vi "K2450 Ramp Current.vi"() -> ()   [LabVIEW 2025]
doc: "Author: Scott Hannahs <sth@magnet.fsu.edu>\n\nThis software is licensed for use under the “MIT License\"\nCopyright (c) 2025 Scott Hannahs, sth@sth@magnet.sthnet.net\n\nPermission is hereby granted, free of charge, to any person obtaining a copy of this software and associated documentation files (the \"Software\"), to deal in the Software without restriction, including without limitation the rights to use, copy, modify, merge, publish, distribute, sublicense, and/or sell copies of the Software, and to permit persons to whom the Software is furnished to do so, subject to the following conditions: The above copyright notice and this permission notice shall be included in all copies or substantial portions of the Software.\n\nTHE SOFTWARE IS PROVIDED \"AS IS\", WITHOUT WARRANTY OF ANY KIND, EXPRESS OR IMPLIED, INCLUDING BUT NOT LIMITED TO THE WARRANTIES OF MERCHANTABILITY, FITNESS FOR A PARTICULAR PURPOSE AND NONINFRINGEMENT. IN NO EVENT SHALL THE AUTHORS OR COPYRIGHT HOLDERS BE LIABLE FOR ANY CLAIM, DAMAGES OR OTHER LIABILITY, WHETHER IN AN ACTION OF CONTRACT, TORT OR OTHERWISE, ARISING FROM, OUT OF OR IN CONNECTION WITH THE SOFTWARE OR THE USE OR OTHER DEALINGS IN THE SOFTWARE."
panel:
  out "Time Remaining":dbl=60.0 format="%<%H:%M:%S>t"
  out "Output Current":dbl format="%_4g"
  in  "Time (Hr:Min:Sec)":dbl=60.0 step=1.0 format="%<%H:%M:%S>t"
  in  "Stop Current":dbl=0.01 format="%_4g"
  in  "Start Ramp":bool
  in  "Cycle Time":dbl=0.1 format="%.3g"
  in  "stop":bool
  in  "VISA resource name":refnum<visa-resource-name>
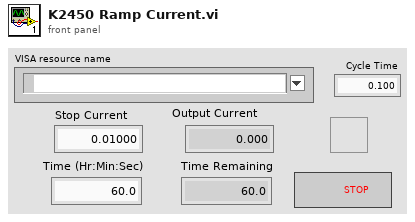
[diagram p1: front panel]
types:
  T1 = enum8{"Enabled", "Disabled", "Disabled and Grayed Out"}
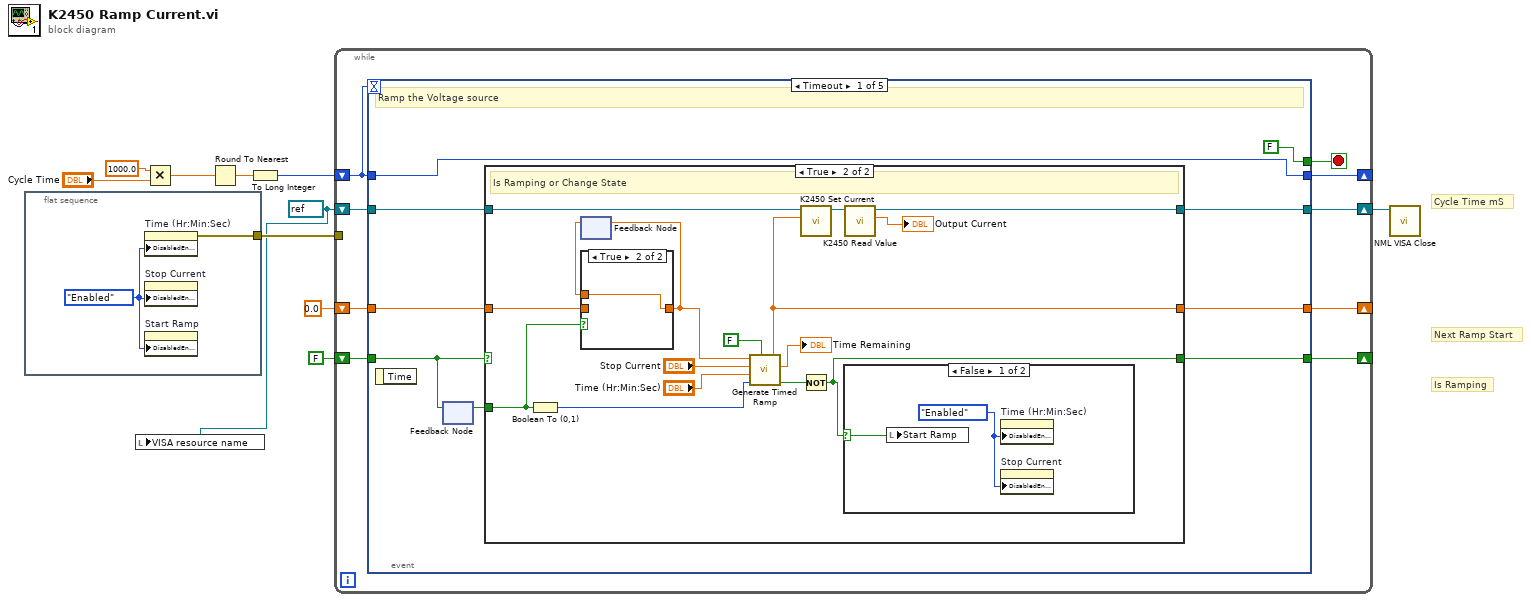
[diagram p0: block diagram]
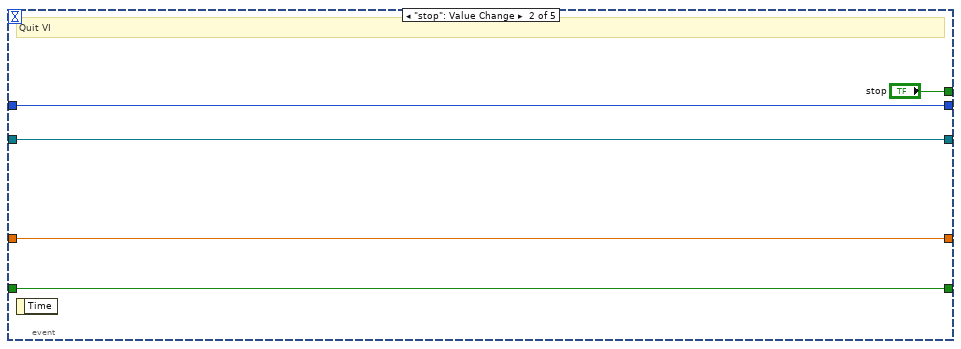
[diagram p5: hidden frame]
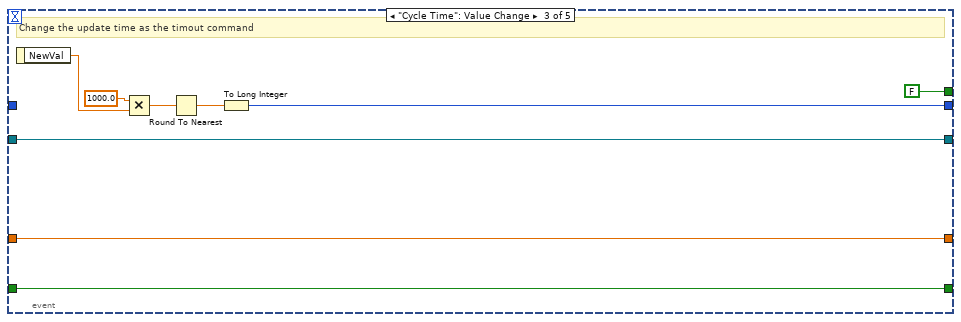
[diagram p6: hidden frame]
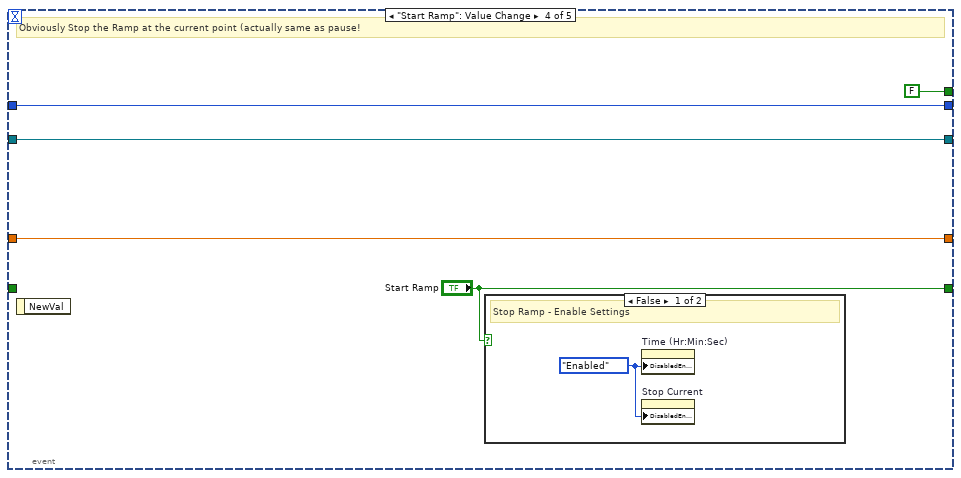
[diagram p7: hidden frame]
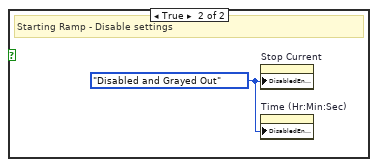
[diagram p8: hidden frame]
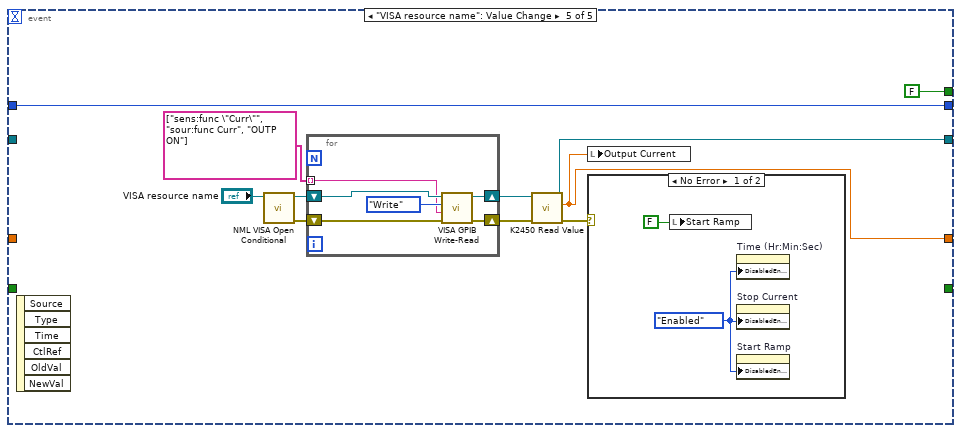
[diagram p9: hidden frame]
diagram:
  w1 = refnum<visa-resource-name> refnum ("dup VISA Session")
  # "Is Ramping"
  # "Next Ramp Start"
  # "Cycle Time mS"
  n1 = flat-sequence {
    tunnel: [w11] -> w2
    frame #0 {
      w12 = T1."Enabled" ("Disabled")
      n2 = property on="Time (Hr:Min:Sec)" class="DigNum (strict)"("DisabledEnum"=w12) -> (error out=w11:errorcluster)  [unwired: 2 in, 1 out]
      n3 = property on="Stop Current" class="DigNum (strict)"("DisabledEnum"=w12) -> ()  [unwired: 2 in, 2 out]
      n4 = property on="Start Ramp" class="Bool (strict)"("DisabledEnum"=w12) -> ()  [unwired: 2 in, 2 out]
    }
  }
  n5 = local write "VISA resource name"(w1) -> ()
  n6 = Multiply(x=1000.0, y="Cycle Time") -> (x*y=w9:dbl)
  n7 = Round To Nearest(number=w9) -> (nearest integer value=w7:dbl)
  n8 = To Long Integer(number=w7) -> (32bit integer=w6:i32)
  n9 = while {
    shift-right: [w17] -> w5
    shift-left: w1 -> [w18]
    shift-right: [w14] -> _
    shift-left: 0.0 ("Voitage 2450") -> [w13]
    shift-right: [w19] -> _
    shift-left: w6 -> [w20]
    shift-right: [w15] -> _
    shift-left: FALSE -> [w16]
    tunnel: w2 -> [_]
    stop <- w21 stop-if-true
    n10 = event shown="[0] Timeout" {
      selector: _ -> [_ _ _ _ _]
      dyn-events: _ -> [_ _ _ _ _]
      timeout: w20 -> [_ _ _ _ _]
      tunnel: [FALSE ("stop") "stop" FALSE ("stop") FALSE ("stop") FALSE ("stop")] -> w21
      tunnel: w20 -> [w30 w57 _ w71 w78]
      tunnel: [w30 w57 w63 w71 w78] -> w19
      tunnel: w18 -> [w29 w54 w60 w70 _]
      tunnel: [w28 w54 w60 w70 w79] -> w17
      tunnel: w16 -> [w23 w56 w61 _ _]
      tunnel: [w26 w56 w61 "Start Ramp" _] -> w15
      tunnel: [w24 w55 w59 w69 w75] -> w14
      tunnel: w13 -> [w25 w55 w59 w69 _]
      event Timeout {
        # "Ramp the Voltage source"
        n11 = event-data() -> ()  [unwired: 1 in, 1 out]
        n12 = feedback-in #1(w23) -> ()
        n13 = feedback #1() -> (w22:bool)  [unwired: 1 in]
        n14 = case shown="True" w23 {
          selector: w23 -> [w31 _]
          tunnel: w29 -> [w33 w48]
          tunnel: [w33 w35] -> w28
          tunnel: [w31 w42] -> w26
          tunnel: w25 -> [w32 w40]
          tunnel: [w32 w43] -> w24
          tunnel: w22 -> [_ w41]
          frame False {
            # "Idle"
          }
          frame True {
            # "Is Ramping or Change State"
            n15 = Boolean To (0,1)(Boolean=w41) -> (0, 1=w47:i16)
            n16 = feedback #2() -> (w38:dbl)  [unwired: 1 in]
            n17 = case shown="True" w41 {
              tunnel: w40 -> [w50 _]
              tunnel: [w50 w51] -> w39
              tunnel: w38 -> [_ w51]
              frame False {
              }
              frame True {
              }
            }
            n18 = feedback-in #2(w39) -> ()
            n19 = call "Generate Timed Ramp.vi"("Log"=FALSE, "Point #"=w47, "Time (Hr:Min:Sec)"="Time (Hr:Min:Sec)", "Stop"="Stop Current", "Start"=w39) -> ("Stop"=w46:bool, "Time Remaining"=→"Time Remaining":dbl, "Output"=w43:dbl)  [unwired: 1 out]
            n20 = call "K2450 Set Current.vi"("Current 2450"=w43, "VISA resource name"=w48) -> ("dup VISA Session"=w36:refnum<visa-resource-name>)  [unwired: 8 in, 1 out]
            n21 = Not(x=w46) -> (.not. x?=w42:bool)
            n22 = case shown="False" w42 {
              selector: w42 -> [w53 _]
              frame False {
                w52 = T1."Enabled" ("Disabled")
                n23 = local write "Start Ramp"(w53) -> ()
                n24 = property on="Time (Hr:Min:Sec)" class="DigNum (strict)"("DisabledEnum"=w52) -> ()  [unwired: 2 in, 2 out]
                n25 = property on="Stop Current" class="DigNum (strict)"("DisabledEnum"=w52) -> ()  [unwired: 2 in, 2 out]
              }
              frame True {
              }
            }
            n26 = call "K2450 Read Value.vi"("VISA resource name"=w36) -> ("Value 2450"=→"Output Current":dbl, "dup VISA Session"=w35:refnum<visa-resource-name>)  [unwired: 8 in, 1 out]
          }
        }
      }
      event "stop": Value Change {
        # "Quit VI"
        n27 = event-data() -> ()  [unwired: 1 in, 1 out]
      }
      event "Cycle Time": Value Change {
        # "Change the update time as the timout command"
        n28 = event-data() -> ("NewVal"=w64:dbl)  [unwired: 1 in]
        n29 = Multiply(x=1000.0, y=w64) -> (x*y=w65:dbl)
        n30 = Round To Nearest(number=w65) -> (nearest integer value=w67:dbl)
        n31 = To Long Integer(number=w67) -> (32bit integer=w63:i32)
      }
      event "Start Ramp": Value Change {
        # "Obviously Stop the Ramp at the current point (actually same as pause!"
        n32 = event-data() -> ()  [unwired: 1 in, 1 out]
        n33 = case shown="False" "Start Ramp" {
          frame False {
            w73 = T1."Enabled" ("Disabled")
            # "Stop Ramp - Enable Settings"
            n34 = property on="Time (Hr:Min:Sec)" class="DigNum (strict)"("DisabledEnum"=w73) -> ()  [unwired: 2 in, 2 out]
            n35 = property on="Stop Current" class="DigNum (strict)"("DisabledEnum"=w73) -> ()  [unwired: 2 in, 2 out]
          }
          frame True {
            w74 = T1."Disabled and Grayed Out" ("Disabled")
            # "Starting Ramp - Disable settings"
            n36 = property on="Stop Current" class="DigNum (strict)"("DisabledEnum"=w74) -> ()  [unwired: 2 in, 2 out]
            n37 = property on="Time (Hr:Min:Sec)" class="DigNum (strict)"("DisabledEnum"=w74) -> ()  [unwired: 2 in, 2 out]
          }
        }
      }
      event "VISA resource name": Value Change {
        n38 = event-data() -> ()  [unwired: 1 in, 6 out]
        n39 = call "NML VISA Open Conditional.vi"("VISA resource name"="VISA resource name") -> ("error out"=w85:errorcluster, "dup VISA Session"=w82:refnum<visa-resource-name>)  [unwired: 8 in, 1 out]
        n40 = for {
          shift-right: [w91] -> w83
          shift-left: w82 -> [w89]
          shift-right: [w92] -> w84
          shift-left: w85 -> [w90]
          tunnel: string[] ["sens:func \"Curr\"", "sour:func Curr", "OUTP ON"] -> [w88] mode=indexing
          n41 = call "VISA GPIB Write-Read.vi"("error in (no error)"=w90, "Command"=w88, "Action"=enum16{"Write", "Read", "Write & Read"}."Write", "VISA resource name"=w89) -> ("error out"=w92:errorcluster, "dup VISA Session"=w91:refnum<visa-resource-name>)  [unwired: 4 in, 2 out]
        }
        n42 = call "K2450 Read Value.vi"("error in (no error)"=w84, "VISA resource name"=w83) -> ("error out"=w76:errorcluster, "Value 2450"=w75:dbl, "dup VISA Session"=w79:refnum<visa-resource-name>)  [unwired: 7 in]
        n43 = local write "Output Current"(w75) -> ()
        n44 = case shown="No Error" w76 {
          frame No Error {
            w87 = T1."Enabled" ("Disabled")
            n45 = local write "Start Ramp"(FALSE ("Start Ramp")) -> ()
            n46 = property on="Time (Hr:Min:Sec)" class="DigNum (strict)"("DisabledEnum"=w87) -> ()  [unwired: 2 in, 2 out]
            n47 = property on="Stop Current" class="DigNum (strict)"("DisabledEnum"=w87) -> ()  [unwired: 2 in, 2 out]
            n48 = property on="Start Ramp" class="Bool (strict)"("DisabledEnum"=w87) -> ()  [unwired: 2 in, 2 out]
          }
          frame Error {
          }
        }
      }
    }
  }
  n49 = call "NML VISA Close.vi"("VISA resource name"=w5) -> ()  [unwired: 10 in, 1 out]
